vi "Exercises_5-1-2.vi"() -> ()   [LabVIEW 2014]
panel:
  out "Intensity Graph":dbl[][](graph)
  out "Array":dbl[][](array[numeric])
  in  "Colums":i32
  in  "Rows":i32
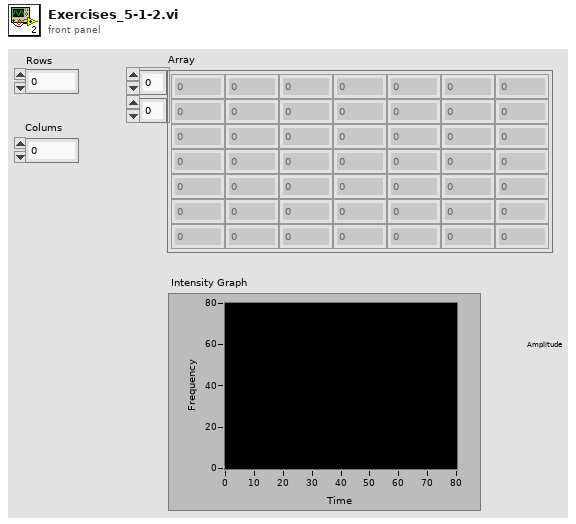
[diagram p1: front panel]
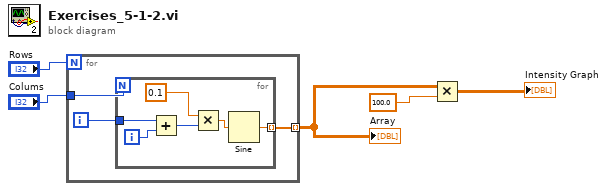
[diagram p0: block diagram]
diagram:
  n1 = for {
    N: "Rows" -> [_]
    tunnel: "Colums" -> [w8]
    tunnel: [w6] -> w2 mode=indexing
    i -> [w7]
    n2 = for {
      N: w8 -> [_]
      tunnel: w7 -> [w14]
      tunnel: [w9] -> w6 mode=indexing
      i -> [w13]
      n3 = Add(x=w14, y=w13) -> (x+y=w11:i32)
      n4 = Multiply(x=0.1, y=w11) -> (x*y=w10:dbl)
      n5 = Sine(x=w10) -> (sin(x)=w9:dbl)
    }
  }
  "Array" <- w2
  n6 = Multiply(x=w2, y=100.0) -> (x*y=→"Intensity Graph":dbl[][])
